vi "Get_SglVar_Value.vi"(8 "error in (no error)":errorcluster, 11 "mupExpr in":refnum<data-value>) -> (0 "error out":errorcluster, 2 "Value":dbl, 3 "mupExpr out":refnum<data-value>)   [LabVIEW 2015, in "mupExpr.lvclass"]
uses:
  mupExpr.lvclass
  mupExpr.lvclass/mupExpr.ctl
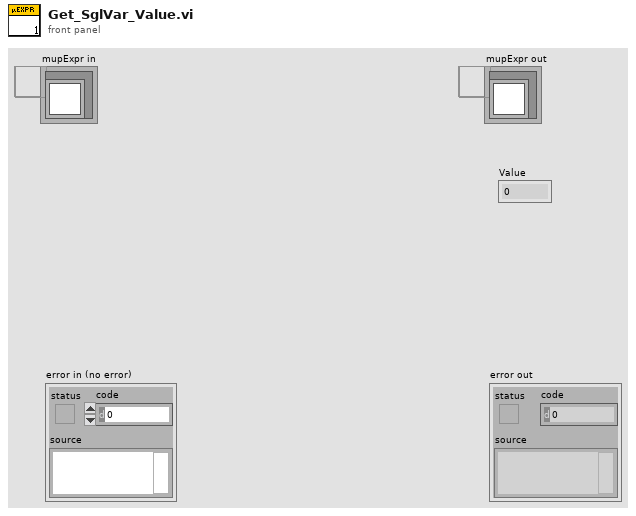
[diagram p1: front panel]
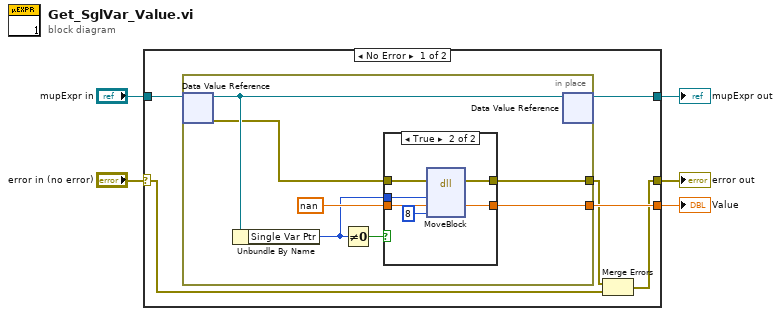
[diagram p0: block diagram]
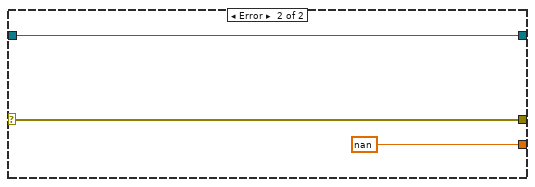
[diagram p3: hidden frame]
diagram:
  n1 = case shown="No Error" "error in (no error)" {
    selector: "error in (no error)" -> [w8 w29]
    tunnel: [w6 w29] -> w4
    tunnel: [w9 w28] -> w2
    tunnel: "mupExpr in" -> [w10 w28]
    tunnel: [w11 nan ("pd")] -> w1
    frame No Error {
      n2 = in-place {
        in-place-border: [w17] -> w7
        in-place-border: [w14] -> w11
        n3 = in-place-dvr #1(w10) -> (w13:refnum<class "mupExpr.lvclass">, w12:errorcluster)
        n4 = Unbundle By Name(w13) -> ("Single Var Ptr"=w16:u64)
        n5 = Not Equal To 0?(x=w16) -> (x != 0?=w15:bool)
        n6 = case shown="True" w15 {
          tunnel: nan ("pd") -> [w19 w25]
          tunnel: w12 -> [w20 w24]
          tunnel: [w20 w23] -> w17
          tunnel: w16 -> [_ w22]
          tunnel: [w19 w21] -> w14
          frame False {
          }
          frame True {
            n7 = dll-call lib="LabVIEW" fn="MoveBlock"(error in=w24, "ps"=w22, "pd"=w25, "size"=8) -> (error out=w23:errorcluster, "pd"=w21:dbl)  [unwired: 5 in, 1 out]
          }
        }
        n8 = in-place-dvr #1(w13) -> (w9:refnum<data-value>)  [unwired: 1 out]
      }
      n9 = Merge Errors(w7, w8) -> (w6:errorcluster)
    }
    frame Error {
    }
  }
  "error out" <- w4
  "mupExpr out" <- w2
  "Value" <- w1
